vi "GenAIChanVarName.vi"(5 "AI Channel":T1) -> (2 "Channel Variable Name":string)   [LabVIEW 2013]
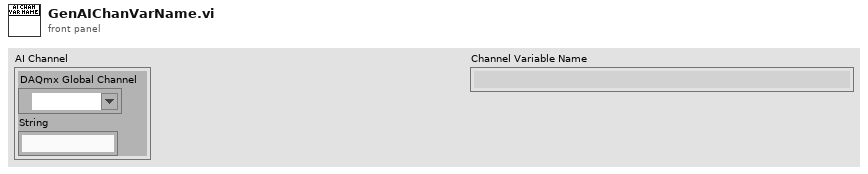
[diagram p1: front panel]
types:
  T1 = cluster{"DAQmx Global Channel":refnum<k21>, "String":string}
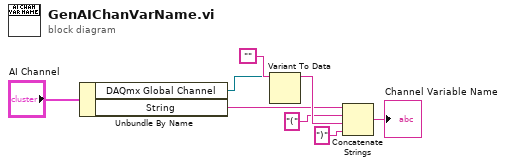
[diagram p0: block diagram]
diagram:
  n1 = Unbundle By Name("AI Channel") -> ("DAQmx Global Channel"=w3:refnum<k21>, "String"=w5:string)
  n2 = Variant To Data(type="", Variant=w3) -> (data=w8:string)  [unwired: 1 in, 1 out]
  n3 = Concatenate Strings(w5, "(" ("string"), w8, ")" ("string")) -> (→"Channel Variable Name":string)
